vi "ADQ Delete ADQ Control Unit (ILYA).vi"(8 "error in (no error)":errorcluster, 11 "adq_cu_ptr":u32) -> (0 "error out":errorcluster, 2 "Error somewhere":bool=TRUE, 3 "adq_cu_ptr out":u32)   [LabVIEW 2013]
doc: "extern \"C\" __declspec(dllimport) void DeleteADQControlUnit(void* adq_cu_ptr);"
uses:
  dlls/ADQAPI.dll
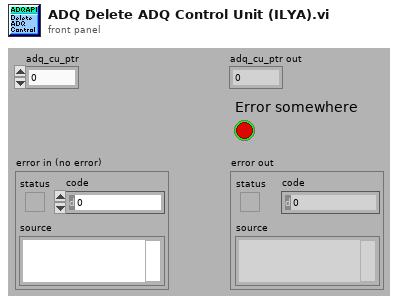
[diagram p1: front panel]
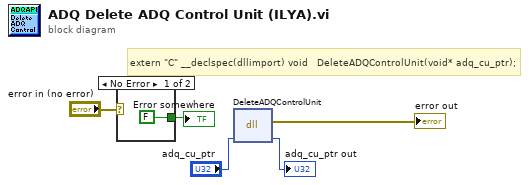
[diagram p0: block diagram]
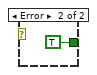
[diagram p2: hidden frame]
diagram:
  # "extern \"C\" __declspec(dllimport) void\t\t\tDeleteADQControlUnit(void* adq_cu_ptr);"
  n1 = case shown="No Error" "error in (no error)" {
    tunnel: [FALSE TRUE] -> w1
    frame No Error {
    }
    frame Error {
    }
  }
  "Error somewhere" <- w1
  n2 = dll-call lib="C:/Users/astafiev/Desktop/IlyaDrive/@photonCounting/LabView_Imperium/dlls/ADQAPI.*" fn="DeleteADQControlUnit"("adq_cu_ptr"="adq_cu_ptr") -> (error out=→"error out":errorcluster, "adq_cu_ptr"=→"adq_cu_ptr out":u32)  [unwired: 4 in, 1 out]
